vi "Lab 4buffered.vi"() -> ()   [LabVIEW 2010]
panel:
  out "ErrCode 2":i32
  out "ErrMsg 2":string
  out "Waveform Graph":u16[](graph)
  in  "LowChan":i32
  in  "HighChan":i32
  in  "InterChannel Delay":sgl=-1.0 format="%.2f"
  in  "Count":i32
  in  "Rate":i32
  in  "Range":i32(ring)=2 items=["Not Programmable"=0, "+- 20 V"=27, "+- 10 V"=1, "+- 5 V"=2, "+- 4 V"=28, "+- 2.5 V"=3, "+- 2 V"=29, "+- 1.67 V"=4, "+- 1.25 V"=5, "+- 1 V"=6, "+- .625 V"=7, "+- .5 V"=8, "+- .25 V"=30, "+- .2 V"=31, "+- .1 V"=9, "+- .05 V"=10, "+- .01 V"=11, "+- .005 V"=12, "0 - 10 V"=13, "0 - 5 V"=14, "0 - 4 V"=36, "0 - 2.5 V"=15, "0 - 2 V"=16, "0 - 1.67 V"=17, "0 - 1.25 V"=18, "0 - 1 V"=19, "0 - .5 V"=32, "0 - .25 V"=33, "0 - .2 V"=34, "0 - .1 V"=20, "0 - .02 V"=35, "0 - .01 V"=21, "4 - 20 mA"=22, "2 - 10 mA"=23, "1 - 5 mA"=24, ".5 - 2.5 mA"=25, "0 - 20 mA"=26]
  in  "Options":i32
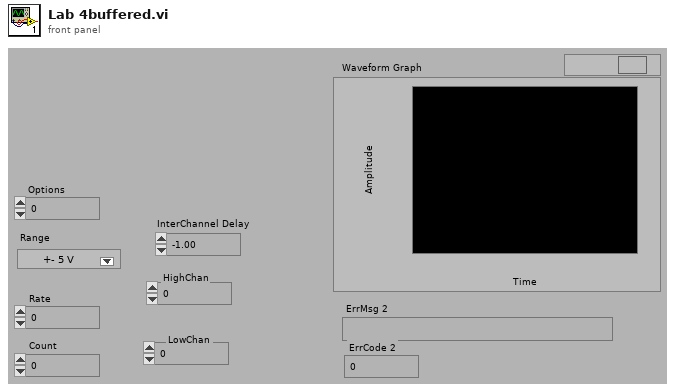
[diagram p1: front panel]
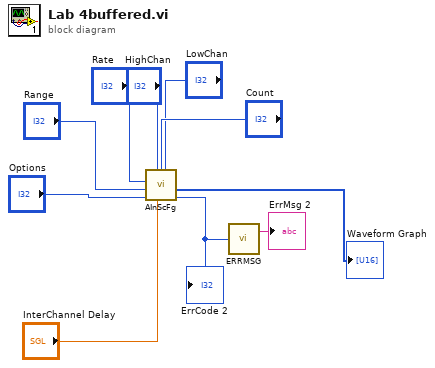
[diagram p0: block diagram]
diagram:
  n1 = call <menus>:"AInScFg.VI"("LowChan"="LowChan", "InterChannel Delay"="InterChannel Delay", "HighChan"="HighChan", "Options"="Options", "Range"="Range", "Rate"="Rate", "Count"="Count") -> ("ErrCode"=w1:i32, "ADData"=→"Waveform Graph":u16[])  [unwired: 1 in, 1 out]
  "ErrCode 2" <- w1
  n2 = call <menus>:"ERRMSG.VI"("ErrCode"=w1) -> ("ErrMsg"=→"ErrMsg 2":string)  [unwired: 1 out]
